vi "Configure_All SMUs_Manual.vi"(7 "HV and PI<0> Settings":T4={"HV SMU Settings"={"Source Range"=30.0, "Source Limit"=1e-05, "Source  limit range"=0.0001, "Source level"=60.0, "CH"="0", "Output Enabled"=FALSE, "Source Mode"=enum."Current", "aperture time"=0.001, "sense 2"=1009}, "PI<0>"={"Source Range"=6.0, "Source Limit"=0.01, "Source  limit range"=0.01, "Source level"=1.2, "CH"="0", "Output Enabled"=FALSE, "Source Mode"=enum."Voltage", "aperture time"=0.01666, "sense 2"=1009}} {"PI<0>"."sense 2" items=["Local"=1008, "Remote"=1009]; "PI<0>"."aperture time" format="%#_13p"; "PI<0>"."Source level" format="%#.6p"; "PI<0>"."Source  limit range" format="%#.6p"; "PI<0>"."Source Limit" format="%#.6p"; "PI<0>"."Source Range" format="%#.6p"; "HV SMU Settings"."sense 2" items=["Local"=1008, "Remote"=1009]; "HV SMU Settings"."aperture time" format="%#_13p"; "HV SMU Settings"."Source level" format="%#.6p"; "HV SMU Settings"."Source  limit range" format="%#.6p"; "HV SMU Settings"."Source Limit" format="%#.6p"; "HV SMU Settings"."Source Range" format="%#.6p"}, 8 "Error In":errorcluster, 10 "DUT and Bridge SMU Settings":T5={"SMU Settings"={"CH"={"voltage level range"=6.0, "current limit"=0.1, "current limit range"=0.1, "voltage level "=1.2, "CH"="0", "Output Enabled"=FALSE}, "CH 2"={"voltage level range"=6.0, "current limit"=0.001, "current limit range"=0.001, "voltage level "=5.0, "CH"="1", "Output Enabled"=FALSE}, "CH 3"={"voltage level range"=6.0, "current limit"=0.001, "current limit range"=0.001, "voltage level "=-5.0, "CH"="2", "Output Enabled"=FALSE}, "CH 4"={"voltage level range"=6.0, "current limit"=0.01, "current limit range"=0.01, "voltage level "=1.8, "CH"="3", "Output Enabled"=FALSE}}, "sense"=1008, "aperture time"=0.01666} {"aperture time" format="%.2p"; "sense" items=["Local"=1008, "Remote"=1009]; "SMU Settings"."CH 4"."voltage level" format="%#.6p"; "SMU Settings"."CH 4"."current limit range" format="%#.6p"; "SMU Settings"."CH 4"."current limit" format="%#.6p"; "SMU Settings"."CH 4"."voltage level range" format="%#.6p"; "SMU Settings"."CH 3"."voltage level" format="%#.6p"; "SMU Settings"."CH 3"."current limit range" format="%#.6p"; "SMU Settings"."CH 3"."current limit" format="%#.6p"; "SMU Settings"."CH 3"."voltage level range" format="%#.6p"; "SMU Settings"."CH 2"."voltage level" format="%#.6p"; "SMU Settings"."CH 2"."current limit range" format="%#.6p"; "SMU Settings"."CH 2"."current limit" format="%#.6p"; "SMU Settings"."CH 2"."voltage level range" format="%#.6p"; "SMU Settings"."CH"."voltage level" format="%#.6p"; "SMU Settings"."CH"."current limit range" format="%#.6p"; "SMU Settings"."CH"."current limit" format="%#.6p"; "SMU Settings"."CH"."voltage level range" format="%#.6p"}, 11 "Instrument_Visas":T6) -> (0 "Error Out":errorcluster, 2 "4_CH_SMu":T2(array[cluster]) {"sense 2" items=["Local"=1008, "Remote"=1009]}, 3 "HV and PI<0> Instrument Settings Readback":T3={"HV SMU Settings: Readback"={"Source Range"=6.0, "Source Limit"=0.01, "Source  limit range"=0.01, "Source level"=1.2, "CH"="0", "Output Enabled"=FALSE, "Source Mode"=enum."Voltage", "aperture time"=0.01666, "sense 2"=1009}, "PI<0>: Settings Readback"={"Source Range"=6.0, "Source Limit"=0.01, "Source  limit range"=0.01, "Source level"=1.2, "CH"="0", "Output Enabled"=FALSE, "Source Mode"=enum."Voltage", "aperture time"=0.01666, "sense 2"=1009}} {"PI<0>: Settings Readback"."sense 2" items=["Local"=1008, "Remote"=1009]; "PI<0>: Settings Readback"."aperture time" format="%#_13p"; "PI<0>: Settings Readback"."Source level" format="%#.6p"; "PI<0>: Settings Readback"."Source  limit range" format="%#.6p"; "PI<0>: Settings Readback"."Source Limit" format="%#.6p"; "PI<0>: Settings Readback"."Source Range" format="%#.6p"; "HV SMU Settings: Readback"."sense 2" items=["Local"=1008, "Remote"=1009]; "HV SMU Settings: Readback"."aperture time" format="%#_13p"; "HV SMU Settings: Readback"."Source level" format="%#.6p"; "HV SMU Settings: Readback"."Source  limit range" format="%#.6p"; "HV SMU Settings: Readback"."Source Limit" format="%#.6p"; "HV SMU Settings: Readback"."Source Range" format="%#.6p"})   [LabVIEW 2013]
uses:
  <instrlib>/niDCPower/nidcpower.llb/niDCPower Sense.ctl
  <instrlib>/niDCPower/nidcpower.llb/niDCPower Aperture Time Units.ctl
  <instrlib>/niDCPower/nidcpower.llb/niDCPower Output Function.ctl
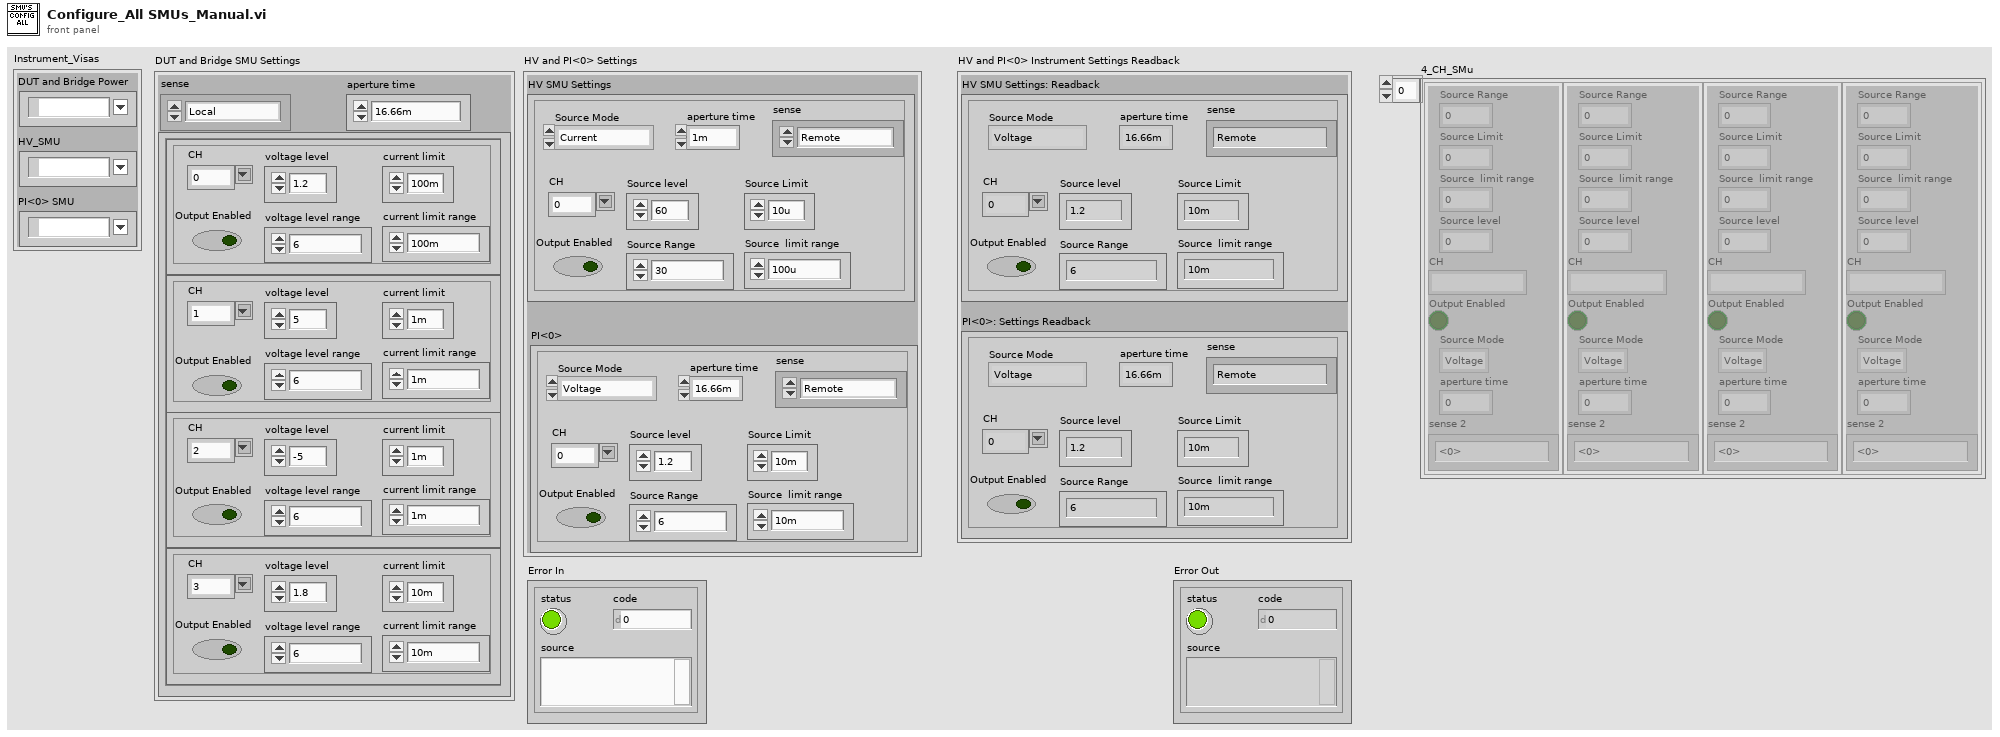
[diagram p1: front panel]
types:
  T1 = typedef "niDCPower Sense.ctl" = i32
  T2 = cluster{"Source Range":dbl, "Source Limit":dbl, "Source  limit range":dbl, "Source level":dbl, "CH":string, "Output Enabled":bool, "Source Mode":enum16{"Voltage", "Current"}, "aperture time":dbl, "sense 2":T1}[]
  T3 = cluster{"HV SMU Settings: Readback":cluster{"Source Range":dbl, "Source Limit":dbl, "Source  limit range":dbl, "Source level":dbl, "CH":string, "Output Enabled":bool, "Source Mode":enum16{"Voltage", "Current"}, "aperture time":dbl, "sense 2":T1}, "PI<0>: Settings Readback":cluster{"Source Range":dbl, "Source Limit":dbl, "Source  limit range":dbl, "Source level":dbl, "CH":string, "Output Enabled":bool, "Source Mode":enum16{"Voltage", "Current"}, "aperture time":dbl, "sense 2":T1}}
  T4 = cluster{"HV SMU Settings":cluster{"Source Range":dbl, "Source Limit":dbl, "Source  limit range":dbl, "Source level":dbl, "CH":string, "Output Enabled":bool, "Source Mode":enum16{"Voltage", "Current"}, "aperture time":dbl, "sense 2":T1}, "PI<0>":cluster{"Source Range":dbl, "Source Limit":dbl, "Source  limit range":dbl, "Source level":dbl, "CH":string, "Output Enabled":bool, "Source Mode":enum16{"Voltage", "Current"}, "aperture time":dbl, "sense 2":T1}}
  T5 = cluster{"SMU Settings":cluster{"CH":cluster{"voltage level range":dbl, "current limit":dbl, "current limit range":dbl, "voltage level ":dbl, "CH":string, "Output Enabled":bool}, "CH 2":cluster{"voltage level range":dbl, "current limit":dbl, "current limit range":dbl, "voltage level ":dbl, "CH":string, "Output Enabled":bool}, "CH 3":cluster{"voltage level range":dbl, "current limit":dbl, "current limit range":dbl, "voltage level ":dbl, "CH":string, "Output Enabled":bool}, "CH 4":cluster{"voltage level range":dbl, "current limit":dbl, "current limit range":dbl, "voltage level ":dbl, "CH":string, "Output Enabled":bool}}, "sense":T1, "aperture time":dbl}
  T6 = cluster{"DUT and Bridge Power":refnum<k15>, "HV_SMU":refnum<k15>, "PI<0> SMU":refnum<k15>}
  T7 = cluster{"Source Range":dbl, "Source Limit":dbl, "Source  limit range":dbl, "Source level":dbl, "CH":string, "Output Enabled":bool, "Source Mode":enum16{"Voltage", "Current"}, "aperture time":dbl, "sense 2":T1}
  T8 = typedef "niDCPower Aperture Time Units.ctl" = i32
  T9 = cluster{"CH":cluster{"voltage level range":dbl, "current limit":dbl, "current limit range":dbl, "voltage level ":dbl, "CH":string, "Output Enabled":bool}, "CH 2":cluster{"voltage level range":dbl, "current limit":dbl, "current limit range":dbl, "voltage level ":dbl, "CH":string, "Output Enabled":bool}, "CH 3":cluster{"voltage level range":dbl, "current limit":dbl, "current limit range":dbl, "voltage level ":dbl, "CH":string, "Output Enabled":bool}, "CH 4":cluster{"voltage level range":dbl, "current limit":dbl, "current limit range":dbl, "voltage level ":dbl, "CH":string, "Output Enabled":bool}}
  T10 = cluster{"voltage level range":dbl, "current limit":dbl, "current limit range":dbl, "voltage level ":dbl, "CH":string, "Output Enabled":bool}[]
  T11 = typedef "niDCPower Output Function.ctl" = i32
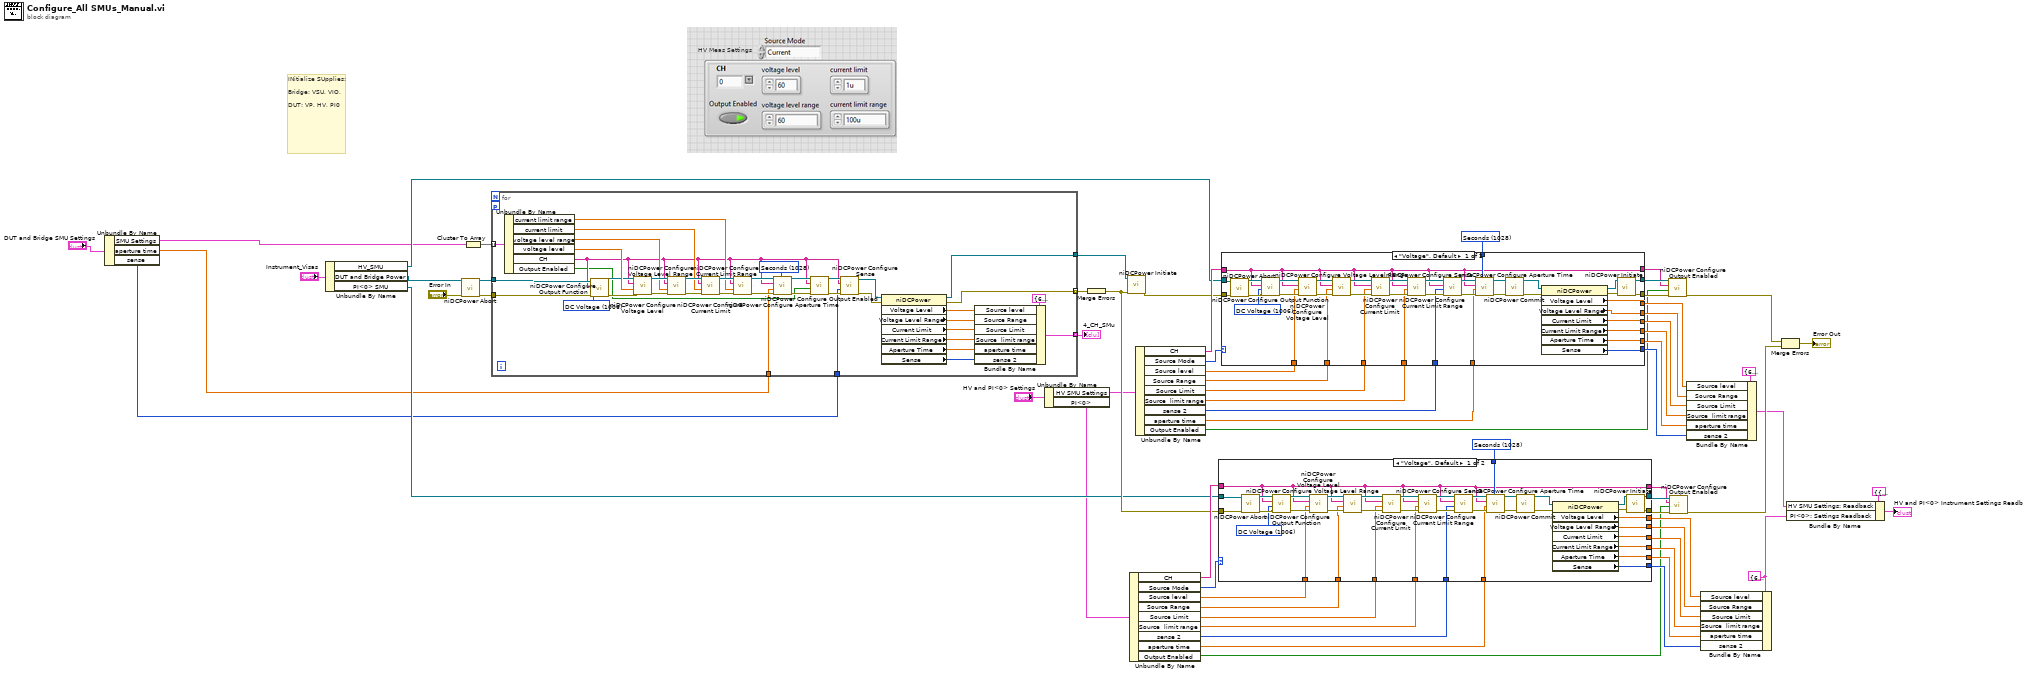
[diagram p0: block diagram]
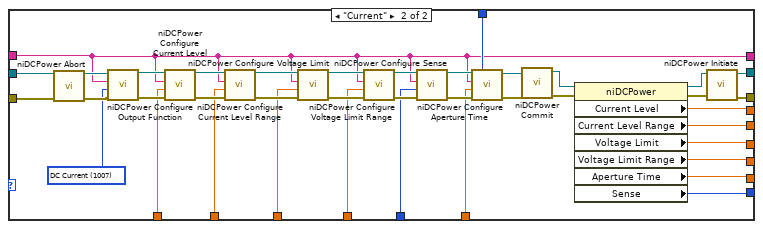
[diagram p2: hidden frame]
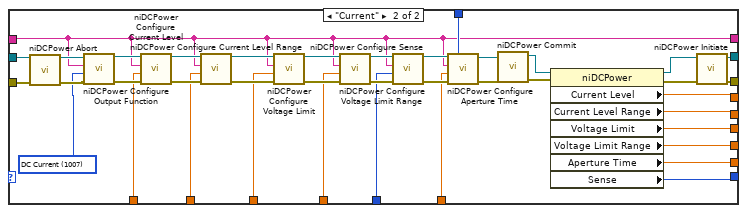
[diagram p3: hidden frame]
diagram:
  w5 = T7 {"Source Range"=6.0, "Source Limit"=0.01, "Source  limit range"=0.01, "Source level"=1.2, "CH"="0", "Output Enabled"=FALSE, "Source Mode"=enum."Voltage", "aperture time"=0.01666, "sense 2"=1009} ("CH 3")
  w44 = T8 1028 items=["Seconds"=1028, "Powerline Cycles"=1029] ("aperture time units")
  w63 = T8 1028 items=["Seconds"=1028, "Powerline Cycles"=1029] ("aperture time units")
  # "HV Meas Settings"
  # "INitialize SUpplies:\n\nBridge: VSU, VIO, \n\nDUT: VP, HV, PI0"
  n1 = Unbundle By Name("DUT and Bridge SMU Settings") -> ("SMU Settings"=w14:T9, "aperture time"=w13:dbl, "sense"=w12:T1)
  n2 = Unbundle By Name("Instrument_Visas") -> ("HV_SMU"=w17:refnum<k15>, "DUT and Bridge Power"=w18:refnum<k15>, "PI<0> SMU"=w16:refnum<k15>)
  n3 = call <instrlib>:"niDCPower Abort.vi"("error in (no error)"="Error In", "instrument handle"=w18) -> ("error out"=w49:errorcluster, "instrument handle out"=w50:refnum<k15>)  [unwired: 8 in]
  n4 = Cluster To Array(cluster=w14) -> (array=w66:T10)
  n5 = for {
    tunnel: w66 -> [w99] mode=indexing
    workers-P: _ -> [_]
    tunnel: w50 -> [w85]
    tunnel: [w76] -> w65
    tunnel: [w68] -> w64 mode=indexing
    tunnel: w49 -> [w83]
    tunnel: w13 -> [w80]
    tunnel: w12 -> [w79]
    tunnel: [w67] -> w1 mode=indexing
    w87 = T11 1006 items=["DC Voltage"=1006, "DC Current"=1007, "Pulse Voltage"=1049, "Pulse Current"=1050] ("output function")
    w88 = T8 1028 items=["Seconds"=1028, "Powerline Cycles"=1029] ("aperture time units")
    n6 = Unbundle By Name(w99) -> ("current limit range"=w95:dbl, "current limit"=w96:dbl, "voltage level range"=w97:dbl, "voltage level"=w98:dbl, "CH"=w82:string, "Output Enabled"=w81:bool)
    n7 = call <instrlib>:"niDCPower Configure Output Function.vi"("error in (no error)"=w83, "output function"=w87, "channel name"=w82, "instrument handle"=w85) -> ("error out"=w86:errorcluster, "instrument handle out"=w84:refnum<k15>)  [unwired: 6 in]
    n8 = call <instrlib>:"niDCPower Configure Voltage Level.vi"("error in (no error)"=w86, "voltage level"=w98, "channel name"=w82, "instrument handle"=w84) -> ("error out"=w104:errorcluster, "instrument handle out"=w105:refnum<k15>)  [unwired: 6 in]
    n9 = call <instrlib>:"niDCPower Configure Voltage Level Range.vi"("error in (no error)"=w104, "voltage level range"=w97, "channel name"=w82, "instrument handle"=w105) -> ("error out"=w103:errorcluster, "instrument handle out"=w102:refnum<k15>)  [unwired: 6 in]
    n10 = call <instrlib>:"niDCPower Configure Current Limit.vi"("error in (no error)"=w103, "current limit"=w96, "channel name"=w82, "instrument handle"=w102) -> ("error out"=w101:errorcluster, "instrument handle out"=w100:refnum<k15>)  [unwired: 6 in]
    n11 = call <instrlib>:"niDCPower Configure Current Limit Range.vi"("error in (no error)"=w101, "current limit range"=w95, "channel name"=w82, "instrument handle"=w100) -> ("error out"=w92:errorcluster, "instrument handle out"=w89:refnum<k15>)  [unwired: 6 in]
    n12 = call <instrlib>:"niDCPower Configure Aperture Time.vi"("aperture time units"=w88, "error in (no error)"=w92, "aperture time"=w80, "channel name"=w82, "instrument handle"=w89) -> ("error out"=w91:errorcluster, "instrument handle out"=w90:refnum<k15>)  [unwired: 5 in]
    n13 = call <instrlib>:"niDCPower Configure Output Enabled.vi"("error in (no error)"=w91, "output enabled"=w81, "channel name"=w82, "instrument handle"=w90) -> ("error out"=w94:errorcluster, "instrument handle out"=w93:refnum<k15>)  [unwired: 6 in]
    n14 = call <instrlib>:"niDCPower Configure Sense.vi"("error in (no error)"=w94, "sense"=w79, "channel name"=w82, "instrument handle"=w93) -> ("error out"=w78:errorcluster, "instrument handle out"=w77:refnum<k15>)  [unwired: 6 in]
    n15 = property class="niDCPower"(reference=w77, error in=w78) -> (reference out=w76:refnum<k15>, error out=w68:errorcluster, "Voltage Level"=w74:dbl, "Voltage Level Range"=w73:dbl, "Current Limit"=w72:dbl, "Current Limit Range"=w71:dbl, "Aperture Time"=w70:dbl, "Sense"=w69:i32)
    n16 = Bundle By Name(cluster=T7 {"Source Range"=6.0, "Source Limit"=0.01, "Source  limit range"=0.01, "Source level"=1.2, "CH"="0", "Output Enabled"=FALSE, "Source Mode"=enum."Voltage", "aperture time"=0.01666, "sense 2"=1009} ("CH 3"), "Source level"=w74, "Source Range"=w73, "Source Limit"=w72, "Source  limit range"=w71, "aperture time"=w70, "sense 2"=w69) -> (w67:T7)
  }
  "4_CH_SMu" <- w1
  n17 = Unbundle By Name("HV and PI<0> Settings") -> ("HV SMU Settings"=w10:T7, "PI<0>"=w9:T7)
  n18 = Merge Errors(w64) -> (w23:errorcluster)
  n19 = call <instrlib>:"niDCPower Initiate.vi"("error in (no error)"=w23, "instrument handle"=w65) -> ("error out"=w2:errorcluster)  [unwired: 8 in, 1 out]
  n20 = Unbundle By Name(w9) -> ("CH"=w24:string, "Source Mode"=w43:enum16{"Voltage", "Current"}, "Source level"=w42:dbl, "Source Range"=w41:dbl, "Source Limit"=w40:dbl, "Source  limit range"=w39:dbl, "sense 2"=w25:T1, "aperture time"=w26:dbl, "Output Enabled"=w20:bool)
  n21 = Unbundle By Name(w10) -> ("CH"=w29:string, "Source Mode"=w62:enum16{"Voltage", "Current"}, "Source level"=w61:dbl, "Source Range"=w60:dbl, "Source Limit"=w59:dbl, "Source  limit range"=w58:dbl, "sense 2"=w27:T1, "aperture time"=w28:dbl, "Output Enabled"=w45:bool)
  n22 = case shown="\"Voltage\", Default" w43 {
    tunnel: [w136 w177] -> w32
    tunnel: [w126 w166] -> w31
    tunnel: w24 -> [w108 w146]
    tunnel: w44 -> [w125 w165]
    tunnel: w26 -> [w124 w164]
    tunnel: w42 -> [w123 w162]
    tunnel: w41 -> [w122 w161]
    tunnel: w40 -> [w121 w160]
    tunnel: w39 -> [w120 w159]
    tunnel: w25 -> [w119 w158]
    tunnel: [w114 w153] -> w38
    tunnel: [w113 w152] -> w37
    tunnel: [w112 w151] -> w36
    tunnel: [w111 w150] -> w35
    tunnel: [w110 w149] -> w34
    tunnel: [w109 w148] -> w33
    tunnel: w16 -> [w106 w147]
    tunnel: [w108 w146] -> w30
    tunnel: w23 -> [w107 w145]
    frame "Voltage", Default {
      w129 = T11 1006 items=["DC Voltage"=1006, "DC Current"=1007, "Pulse Voltage"=1049, "Pulse Current"=1050] ("output function")
      n23 = call <instrlib>:"niDCPower Abort.vi"("error in (no error)"=w107, "instrument handle"=w106) -> ("error out"=w131:errorcluster, "instrument handle out"=w130:refnum<k15>)  [unwired: 8 in]
      n24 = call <instrlib>:"niDCPower Configure Output Function.vi"("error in (no error)"=w131, "output function"=w129, "channel name"=w108, "instrument handle"=w130) -> ("error out"=w127:errorcluster, "instrument handle out"=w128:refnum<k15>)  [unwired: 6 in]
      n25 = call <instrlib>:"niDCPower Configure Voltage Level.vi"("error in (no error)"=w127, "voltage level"=w123, "channel name"=w108, "instrument handle"=w128) -> ("error out"=w144:errorcluster, "instrument handle out"=w143:refnum<k15>)  [unwired: 6 in]
      n26 = call <instrlib>:"niDCPower Configure Voltage Level Range.vi"("error in (no error)"=w144, "voltage level range"=w122, "channel name"=w108, "instrument handle"=w143) -> ("error out"=w142:errorcluster, "instrument handle out"=w140:refnum<k15>)  [unwired: 6 in]
      n27 = call <instrlib>:"niDCPower Configure Current Limit.vi"("error in (no error)"=w142, "current limit"=w121, "channel name"=w108, "instrument handle"=w140) -> ("error out"=w141:errorcluster, "instrument handle out"=w139:refnum<k15>)  [unwired: 6 in]
      n28 = call <instrlib>:"niDCPower Configure Current Limit Range.vi"("error in (no error)"=w141, "current limit range"=w120, "channel name"=w108, "instrument handle"=w139) -> ("error out"=w138:errorcluster, "instrument handle out"=w137:refnum<k15>)  [unwired: 6 in]
      n29 = call <instrlib>:"niDCPower Configure Sense.vi"("error in (no error)"=w138, "sense"=w119, "channel name"=w108, "instrument handle"=w137) -> ("error out"=w135:errorcluster, "instrument handle out"=w134:refnum<k15>)  [unwired: 6 in]
      n30 = call <instrlib>:"niDCPower Configure Aperture Time.vi"("aperture time units"=w125, "error in (no error)"=w135, "aperture time"=w124, "channel name"=w108, "instrument handle"=w134) -> ("error out"=w132:errorcluster, "instrument handle out"=w133:refnum<k15>)  [unwired: 5 in]
      n31 = call <instrlib>:"niDCPower Commit.vi"("error in (no error)"=w132, "instrument handle"=w133) -> ("error out"=w118:errorcluster, "instrument handle out"=w117:refnum<k15>)  [unwired: 8 in]
      n32 = property class="niDCPower"(reference=w117, error in=w118) -> (reference out=w115:refnum<k15>, error out=w116:errorcluster, "Voltage Level"=w114:dbl, "Voltage Level Range"=w113:dbl, "Current Limit"=w112:dbl, "Current Limit Range"=w111:dbl, "Aperture Time"=w110:dbl, "Sense"=w109:i32)
      n33 = call <instrlib>:"niDCPower Initiate.vi"("error in (no error)"=w116, "instrument handle"=w115) -> ("error out"=w136:errorcluster, "instrument handle out"=w126:refnum<k15>)  [unwired: 8 in]
    }
    frame "Current" {
      w169 = T11 1007 items=["DC Voltage"=1006, "DC Current"=1007, "Pulse Voltage"=1049, "Pulse Current"=1050] ("output function")
      n34 = call <instrlib>:"niDCPower Abort.vi"("error in (no error)"=w145, "instrument handle"=w147) -> ("error out"=w171:errorcluster, "instrument handle out"=w170:refnum<k15>)  [unwired: 8 in]
      n35 = call <instrlib>:"niDCPower Configure Output Function.vi"("error in (no error)"=w171, "output function"=w169, "channel name"=w146, "instrument handle"=w170) -> ("error out"=w163:errorcluster, "instrument handle out"=w172:refnum<k15>)  [unwired: 6 in]
      n36 = call <instrlib>:"niDCPower Configure Current Level.vi"("error in (no error)"=w163, "current level"=w162, "channel name"=w146, "instrument handle"=w172) -> ("error out"=w183:errorcluster, "instrument handle out"=w182:refnum<k15>)  [unwired: 6 in]
      n37 = call <instrlib>:"niDCPower Configure Current Level Range.vi"("error in (no error)"=w183, "current level range"=w161, "channel name"=w146, "instrument handle"=w182) -> ("error out"=w181:errorcluster, "instrument handle out"=w180:refnum<k15>)  [unwired: 6 in]
      n38 = call <instrlib>:"niDCPower Configure Voltage Limit.vi"("error in (no error)"=w181, "voltage limit"=w160, "channel name"=w146, "instrument handle"=w180) -> ("error out"=w179:errorcluster, "instrument handle out"=w178:refnum<k15>)  [unwired: 6 in]
      n39 = call <instrlib>:"niDCPower Configure Voltage Limit Range.vi"("error in (no error)"=w179, "voltage limit range"=w159, "channel name"=w146, "instrument handle"=w178) -> ("error out"=w176:errorcluster, "instrument handle out"=w175:refnum<k15>)  [unwired: 6 in]
      n40 = call <instrlib>:"niDCPower Configure Sense.vi"("error in (no error)"=w176, "sense"=w158, "channel name"=w146, "instrument handle"=w175) -> ("error out"=w174:errorcluster, "instrument handle out"=w173:refnum<k15>)  [unwired: 6 in]
      n41 = call <instrlib>:"niDCPower Configure Aperture Time.vi"("aperture time units"=w165, "error in (no error)"=w174, "aperture time"=w164, "channel name"=w146, "instrument handle"=w173) -> ("error out"=w168:errorcluster, "instrument handle out"=w167:refnum<k15>)  [unwired: 5 in]
      n42 = call <instrlib>:"niDCPower Commit.vi"("error in (no error)"=w168, "instrument handle"=w167) -> ("error out"=w157:errorcluster, "instrument handle out"=w156:refnum<k15>)  [unwired: 8 in]
      n43 = property class="niDCPower"(reference=w156, error in=w157) -> (reference out=w154:refnum<k15>, error out=w155:errorcluster, "Current Level"=w153:dbl, "Current Level Range"=w152:dbl, "Voltage Limit"=w151:dbl, "Voltage Limit Range"=w150:dbl, "Aperture Time"=w149:dbl, "Sense"=w148:i32)
      n44 = call <instrlib>:"niDCPower Initiate.vi"("error in (no error)"=w155, "instrument handle"=w154) -> ("error out"=w177:errorcluster, "instrument handle out"=w166:refnum<k15>)  [unwired: 8 in]
    }
  }
  n45 = case shown="\"Voltage\", Default" w62 {
    tunnel: [w214 w255] -> w48
    tunnel: [w204 w244] -> w47
    tunnel: w29 -> [w186 w223]
    tunnel: w63 -> [w203 w243]
    tunnel: w28 -> [w202 w242]
    tunnel: w61 -> [w201 w240]
    tunnel: w60 -> [w200 w239]
    tunnel: w59 -> [w199 w238]
    tunnel: w58 -> [w198 w237]
    tunnel: w27 -> [w197 w236]
    tunnel: [w192 w231] -> w57
    tunnel: [w191 w230] -> w55
    tunnel: [w190 w229] -> w54
    tunnel: [w189 w228] -> w53
    tunnel: [w188 w227] -> w52
    tunnel: [w187 w226] -> w51
    tunnel: w17 -> [w184 w225]
    tunnel: w2 -> [w185 w224]
    tunnel: [w186 w223] -> w46
    frame "Voltage", Default {
      w207 = T11 1006 items=["DC Voltage"=1006, "DC Current"=1007, "Pulse Voltage"=1049, "Pulse Current"=1050] ("output function")
      n46 = call <instrlib>:"niDCPower Abort.vi"("error in (no error)"=w185, "instrument handle"=w184) -> ("error out"=w209:errorcluster, "instrument handle out"=w208:refnum<k15>)  [unwired: 8 in]
      n47 = call <instrlib>:"niDCPower Configure Output Function.vi"("error in (no error)"=w209, "output function"=w207, "channel name"=w186, "instrument handle"=w208) -> ("error out"=w205:errorcluster, "instrument handle out"=w206:refnum<k15>)  [unwired: 6 in]
      n48 = call <instrlib>:"niDCPower Configure Voltage Level.vi"("error in (no error)"=w205, "voltage level"=w201, "channel name"=w186, "instrument handle"=w206) -> ("error out"=w222:errorcluster, "instrument handle out"=w221:refnum<k15>)  [unwired: 6 in]
      n49 = call <instrlib>:"niDCPower Configure Voltage Level Range.vi"("error in (no error)"=w222, "voltage level range"=w200, "channel name"=w186, "instrument handle"=w221) -> ("error out"=w220:errorcluster, "instrument handle out"=w218:refnum<k15>)  [unwired: 6 in]
      n50 = call <instrlib>:"niDCPower Configure Current Limit.vi"("error in (no error)"=w220, "current limit"=w199, "channel name"=w186, "instrument handle"=w218) -> ("error out"=w219:errorcluster, "instrument handle out"=w217:refnum<k15>)  [unwired: 6 in]
      n51 = call <instrlib>:"niDCPower Configure Current Limit Range.vi"("error in (no error)"=w219, "current limit range"=w198, "channel name"=w186, "instrument handle"=w217) -> ("error out"=w216:errorcluster, "instrument handle out"=w215:refnum<k15>)  [unwired: 6 in]
      n52 = call <instrlib>:"niDCPower Configure Sense.vi"("error in (no error)"=w216, "sense"=w197, "channel name"=w186, "instrument handle"=w215) -> ("error out"=w213:errorcluster, "instrument handle out"=w212:refnum<k15>)  [unwired: 6 in]
      n53 = call <instrlib>:"niDCPower Configure Aperture Time.vi"("aperture time units"=w203, "error in (no error)"=w213, "aperture time"=w202, "channel name"=w186, "instrument handle"=w212) -> ("error out"=w210:errorcluster, "instrument handle out"=w211:refnum<k15>)  [unwired: 5 in]
      n54 = call <instrlib>:"niDCPower Commit.vi"("error in (no error)"=w210, "instrument handle"=w211) -> ("error out"=w196:errorcluster, "instrument handle out"=w195:refnum<k15>)  [unwired: 8 in]
      n55 = property class="niDCPower"(reference=w195, error in=w196) -> (reference out=w193:refnum<k15>, error out=w194:errorcluster, "Voltage Level"=w192:dbl, "Voltage Level Range"=w191:dbl, "Current Limit"=w190:dbl, "Current Limit Range"=w189:dbl, "Aperture Time"=w188:dbl, "Sense"=w187:i32)
      n56 = call <instrlib>:"niDCPower Initiate.vi"("error in (no error)"=w194, "instrument handle"=w193) -> ("error out"=w214:errorcluster, "instrument handle out"=w204:refnum<k15>)  [unwired: 8 in]
    }
    frame "Current" {
      w247 = T11 1007 items=["DC Voltage"=1006, "DC Current"=1007, "Pulse Voltage"=1049, "Pulse Current"=1050] ("output function")
      n57 = call <instrlib>:"niDCPower Abort.vi"("error in (no error)"=w224, "instrument handle"=w225) -> ("error out"=w249:errorcluster, "instrument handle out"=w248:refnum<k15>)  [unwired: 8 in]
      n58 = call <instrlib>:"niDCPower Configure Output Function.vi"("error in (no error)"=w249, "output function"=w247, "channel name"=w223, "instrument handle"=w248) -> ("error out"=w241:errorcluster, "instrument handle out"=w250:refnum<k15>)  [unwired: 6 in]
      n59 = call <instrlib>:"niDCPower Configure Current Level.vi"("error in (no error)"=w241, "current level"=w240, "channel name"=w223, "instrument handle"=w250) -> ("error out"=w261:errorcluster, "instrument handle out"=w260:refnum<k15>)  [unwired: 6 in]
      n60 = call <instrlib>:"niDCPower Configure Current Level Range.vi"("error in (no error)"=w261, "current level range"=w239, "channel name"=w223, "instrument handle"=w260) -> ("error out"=w259:errorcluster, "instrument handle out"=w258:refnum<k15>)  [unwired: 6 in]
      n61 = call <instrlib>:"niDCPower Configure Voltage Limit.vi"("error in (no error)"=w259, "voltage limit"=w238, "channel name"=w223, "instrument handle"=w258) -> ("error out"=w257:errorcluster, "instrument handle out"=w256:refnum<k15>)  [unwired: 6 in]
      n62 = call <instrlib>:"niDCPower Configure Voltage Limit Range.vi"("error in (no error)"=w257, "voltage limit range"=w237, "channel name"=w223, "instrument handle"=w256) -> ("error out"=w254:errorcluster, "instrument handle out"=w253:refnum<k15>)  [unwired: 6 in]
      n63 = call <instrlib>:"niDCPower Configure Sense.vi"("error in (no error)"=w254, "sense"=w236, "channel name"=w223, "instrument handle"=w253) -> ("error out"=w252:errorcluster, "instrument handle out"=w251:refnum<k15>)  [unwired: 6 in]
      n64 = call <instrlib>:"niDCPower Configure Aperture Time.vi"("aperture time units"=w243, "error in (no error)"=w252, "aperture time"=w242, "channel name"=w223, "instrument handle"=w251) -> ("error out"=w246:errorcluster, "instrument handle out"=w245:refnum<k15>)  [unwired: 5 in]
      n65 = call <instrlib>:"niDCPower Commit.vi"("error in (no error)"=w246, "instrument handle"=w245) -> ("error out"=w235:errorcluster, "instrument handle out"=w234:refnum<k15>)  [unwired: 8 in]
      n66 = property class="niDCPower"(reference=w234, error in=w235) -> (reference out=w232:refnum<k15>, error out=w233:errorcluster, "Current Level"=w231:dbl, "Current Level Range"=w230:dbl, "Voltage Limit"=w229:dbl, "Voltage Limit Range"=w228:dbl, "Aperture Time"=w227:dbl, "Sense"=w226:i32)
      n67 = call <instrlib>:"niDCPower Initiate.vi"("error in (no error)"=w233, "instrument handle"=w232) -> ("error out"=w255:errorcluster, "instrument handle out"=w244:refnum<k15>)  [unwired: 8 in]
    }
  }
  n68 = call <instrlib>:"niDCPower Configure Output Enabled.vi"("error in (no error)"=w48, "output enabled"=w45, "channel name"=w46, "instrument handle"=w47) -> ("error out"=w22:errorcluster)  [unwired: 6 in, 1 out]
  n69 = call <instrlib>:"niDCPower Configure Output Enabled.vi"("error in (no error)"=w32, "output enabled"=w20, "channel name"=w30, "instrument handle"=w31) -> ("error out"=w21:errorcluster)  [unwired: 6 in, 1 out]
  n70 = Bundle By Name(cluster=T7 {"Source Range"=6.0, "Source Limit"=0.01, "Source  limit range"=0.01, "Source level"=1.2, "CH"="0", "Output Enabled"=FALSE, "Source Mode"=enum."Voltage", "aperture time"=0.01666, "sense 2"=1009} ("CH 3"), "Source level"=w57, "Source Range"=w55, "Source Limit"=w54, "Source  limit range"=w53, "aperture time"=w52, "sense 2"=w51) -> (w6:T7)
  n71 = Bundle By Name(cluster=w5, "Source level"=w38, "Source Range"=w37, "Source Limit"=w36, "Source  limit range"=w35, "aperture time"=w34, "sense 2"=w33) -> ()  [unwired: 1 out]
  n72 = Merge Errors(w22, w21) -> (→"Error Out":errorcluster)
  n73 = Bundle By Name(cluster=T3 {"HV SMU Settings: Readback"={"Source Range"=6.0, "Source Limit"=0.01, "Source  limit range"=0.01, "Source level"=1.2, "CH"="0", "Output Enabled"=FALSE, "Source Mode"=enum."Voltage", "aperture time"=0.01666, "sense 2"=1009}, "PI<0>: Settings Readback"={"Source Range"=6.0, "Source Limit"=0.01, "Source  limit range"=0.01, "Source level"=1.2, "CH"="0", "Output Enabled"=FALSE, "Source Mode"=enum."Voltage", "aperture time"=0.01666, "sense 2"=1009}} ("Cluster 3"), "HV SMU Settings: Readback"=w6, "PI<0>: Settings Readback"=w5) -> (→"HV and PI<0> Instrument Settings Readback":T3)
